vi "Set INI Refnum.vi"(11 "INI Refnum In":T1) -> ()   [LabVIEW 2014, in "Standard Editor.lvlib" / "DCAF INI.lvlib"]
doc: "Set the INI reference of fgv_DCAF INI Refnum.vi"
uses:
  DCAF INI.lvlib
  <vilib>/Utility/config.llb/Config Data RefNum.ctl
  enum_DCAF INI FGV Action.ctl
  <vilib>/Utility/config.llb/NI_LVConfig.lvlib
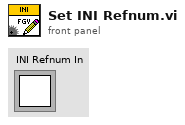
[diagram p1: front panel]
types:
  T1 = typedef "NI_LVConfig.lvlib/Config Data RefNum.ctl" = refnum<k1>
  T2 = typedef "Standard Editor.lvlib/DCAF INI.lvlib/enum_DCAF INI FGV Action.ctl" = enum16{"Get", "Set"}
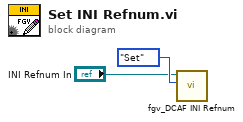
[diagram p0: block diagram]
diagram:
  n1 = call "fgv_DCAF INI Refnum.vi"("Action"=enum_DCAF_INI_FGV_Action."Set", "INI Refnum In"="INI Refnum In") -> ()  [unwired: 9 in, 1 out]
